vi "CSIRO XYZ Target Stage Control.vi"() -> ()   [LabVIEW 2018]
uses:
  PerformaxLV_v103.llb/commandsnew.ctl
  HYMOD MAIA/GLOBAL XYZ STAGE POSITION.vi
  Microdaq FPGA Development/USB XYZ Stage Reference.vi
panel:
  out "read_string 6":string
  out "read_string 5":string
  out "read_string 4":string
  out "DIVERGENCE 2":i32
  in  "Tab Control 3":T1(tab)=enum."CAL"
  in  "ENABLE MOTORS":bool
  in  "SPEED":i32(ring) items=["FAST", "NORMAL", "SLOW", "VERY SLOW", "ULTRASLOW"]
  in  "SET ZERO":bool
  out "Z":dbl[unit]=5.5500255e-05 caption="OY" format="%_6f"
  out "X":dbl[unit]=4.4501529999999996e-05 format="%_6f"
  out "Y":dbl[unit]=5.550153e-05 caption="OY" format="%_6f"
  in  "OY +":bool
  in  "OX -":bool
  in  "OX+":bool
  in  "OY-":bool
  in  "STOP":bool
  out "Y 2":bool
  out "X 2":bool
  out "Z":bool
  in  "DEFINED OBJECT":bool=TRUE
  in  "DEFINED LOCATIONS":i32(ring) items=["GLASS", "2000 CU GRID", "PHOSPHORUS", "5mm Aperture", "OPEN"]
  out "CURRENT LOCATION":string
  out "Z ENC":i32=1
  in  "Y B":dbl[unit] format="%_5f"
  in  "Y A":dbl[unit]=6.950000000000002e-08 format="%#_4f"
  in  "X B":dbl[unit] format="%_5f"
  in  "X A":dbl[unit]=6.950000000000001e-08 format="%#_4f"
  in  "MOVE OBJECT":T2 {"Z" format="%#_5f"; "Y" format="%#_5f"; "X" format="%#_5f"}
  in  "MOVE OBJECTS":bool
  out "X ENC":i32=6
  out "Y ENC":i32=6
  in  "Z A":dbl[unit]=2.5e-07 format="%#_4f"
  in  "Z B":dbl[unit] format="%_5f"
  in  "LOCATIONARRAY":T3(array[cluster])=[{"X"=0.063, "Y"=0.063, "DEFINITION"="0-1mm Object"}, {"X"=0.07602, "Y"=0.08773, "DEFINITION"="1mm Object"}, {"X"=0.08789, "Y"=0.07540000000000001, "DEFINITION"="2mm Object"}, {"X"=0.08789, "Y"=0.08773, "DEFINITION"="5mm Object"}, {"X"=0.12, "Y"=0.12, "DEFINITION"="10mm Object"}, {"X"=0.12, "Y"=0.10073, "DEFINITION"="OUT"}] {"Y" format="%#_4f"; "X" format="%#_4f"}
  in  "OHSPEED":i32=2000 min=1 max=400000 step=1
  in  "OLSPEED":i32=200 min=100 max=490550
  in  "OXACC":i32=300 min=1 max=5000
  in  "OYACC":i32=300 min=1 max=5000
  # "STOP"
  # "Calibration of Motor Positions"
  # "Aperture = A*enc step + B (mm)"
  # "NOTE: 1enc step = 2.5 * motor step"
  # "centre = red dot near 2nd thru hole\ngrid = +5mm (right), +15mm (up)\nsci = +8mm (right),  +13mm (up)\nglass =  +8mm (right), 0mm (up)"
  # "Speed Settings (pps)"
  # "Acceleration (ms)"
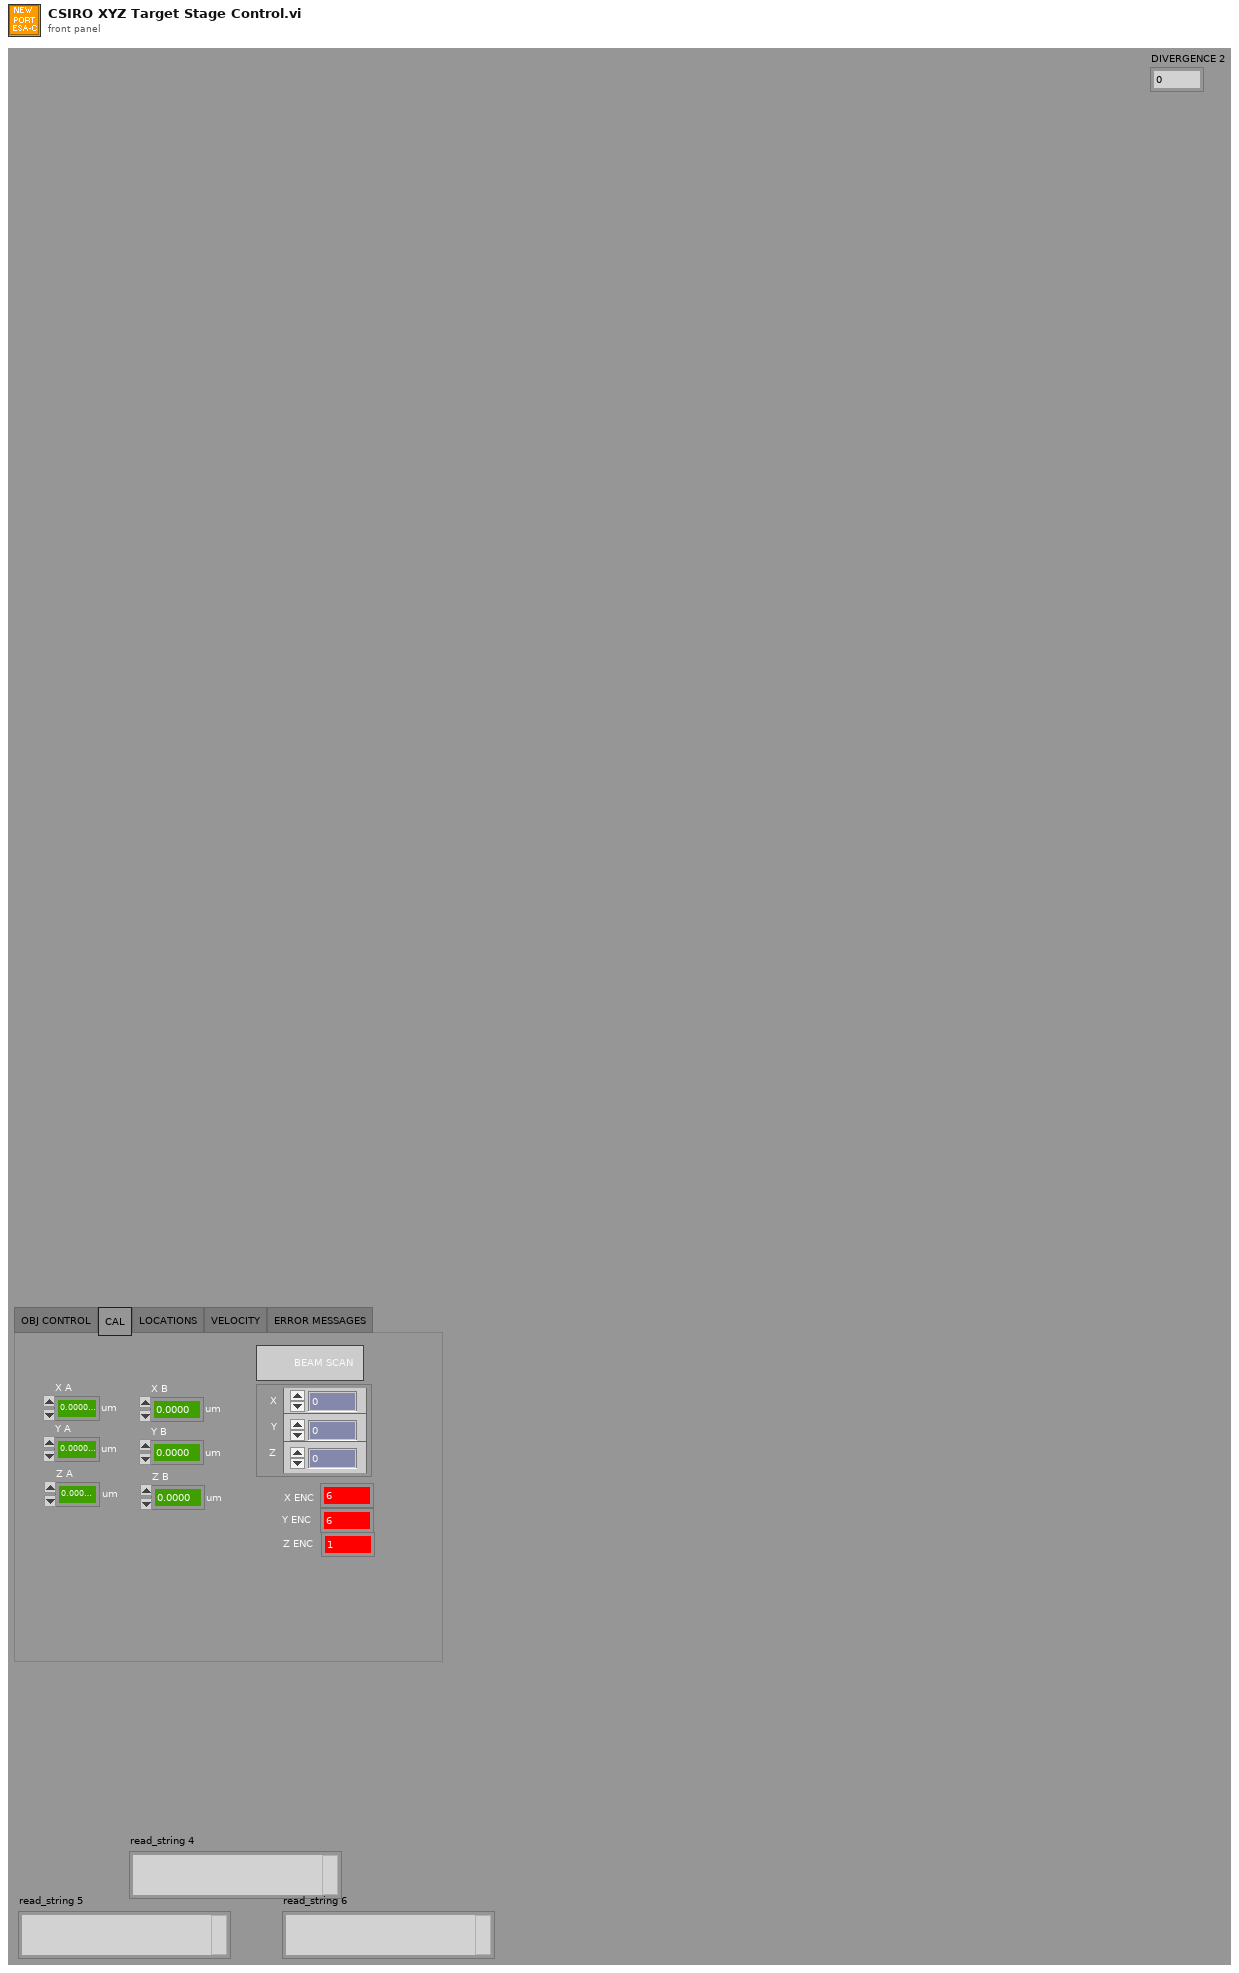
[diagram p1: front panel]
types:
  T1 = enum32{"OBJ CONTROL", "CAL", "LOCATIONS", "VELOCITY", "ERROR MESSAGES"}
  T2 = cluster{"X":dbl[unit], "Y":dbl[unit], "Z":dbl[unit]}
  T3 = cluster{"X":dbl[unit], "Y":dbl[unit], "DEFINITION":string}[]
  T4 = typedef "commandsnew.ctl" = enum16{"clearErr", "constJogNeg", "constJogPos", "getAccel", "getDeviceId", "getFirmwareVer", "getHighSpeed", "getIdleAmp", "getLowSpeed", "getMicroStep", "getMotorStatus", "getPolarity", "getPosition", "getProdId", "getPwrStatus", "getRunAmp", "getStatus", "getTemp", "homeNeg", "homePos", "moveToPosition", "powerDown", "powerUp", "setAccel", "setDeviceId", "setHighSpeed", "setIdleAmp", "setLowSpeed", "setMicroStep", "setPolarityLow", "setPolarityHigh", "setPosition", "setRunAmp", "stopFast", "stopSlow"}
  T5 = cluster{"X":dbl[unit], "Y":dbl[unit], "DEFINITION":string}
  T6 = cluster{"X":dbl[unit], "Y":dbl[unit], "CURRENT LOCATION":string}
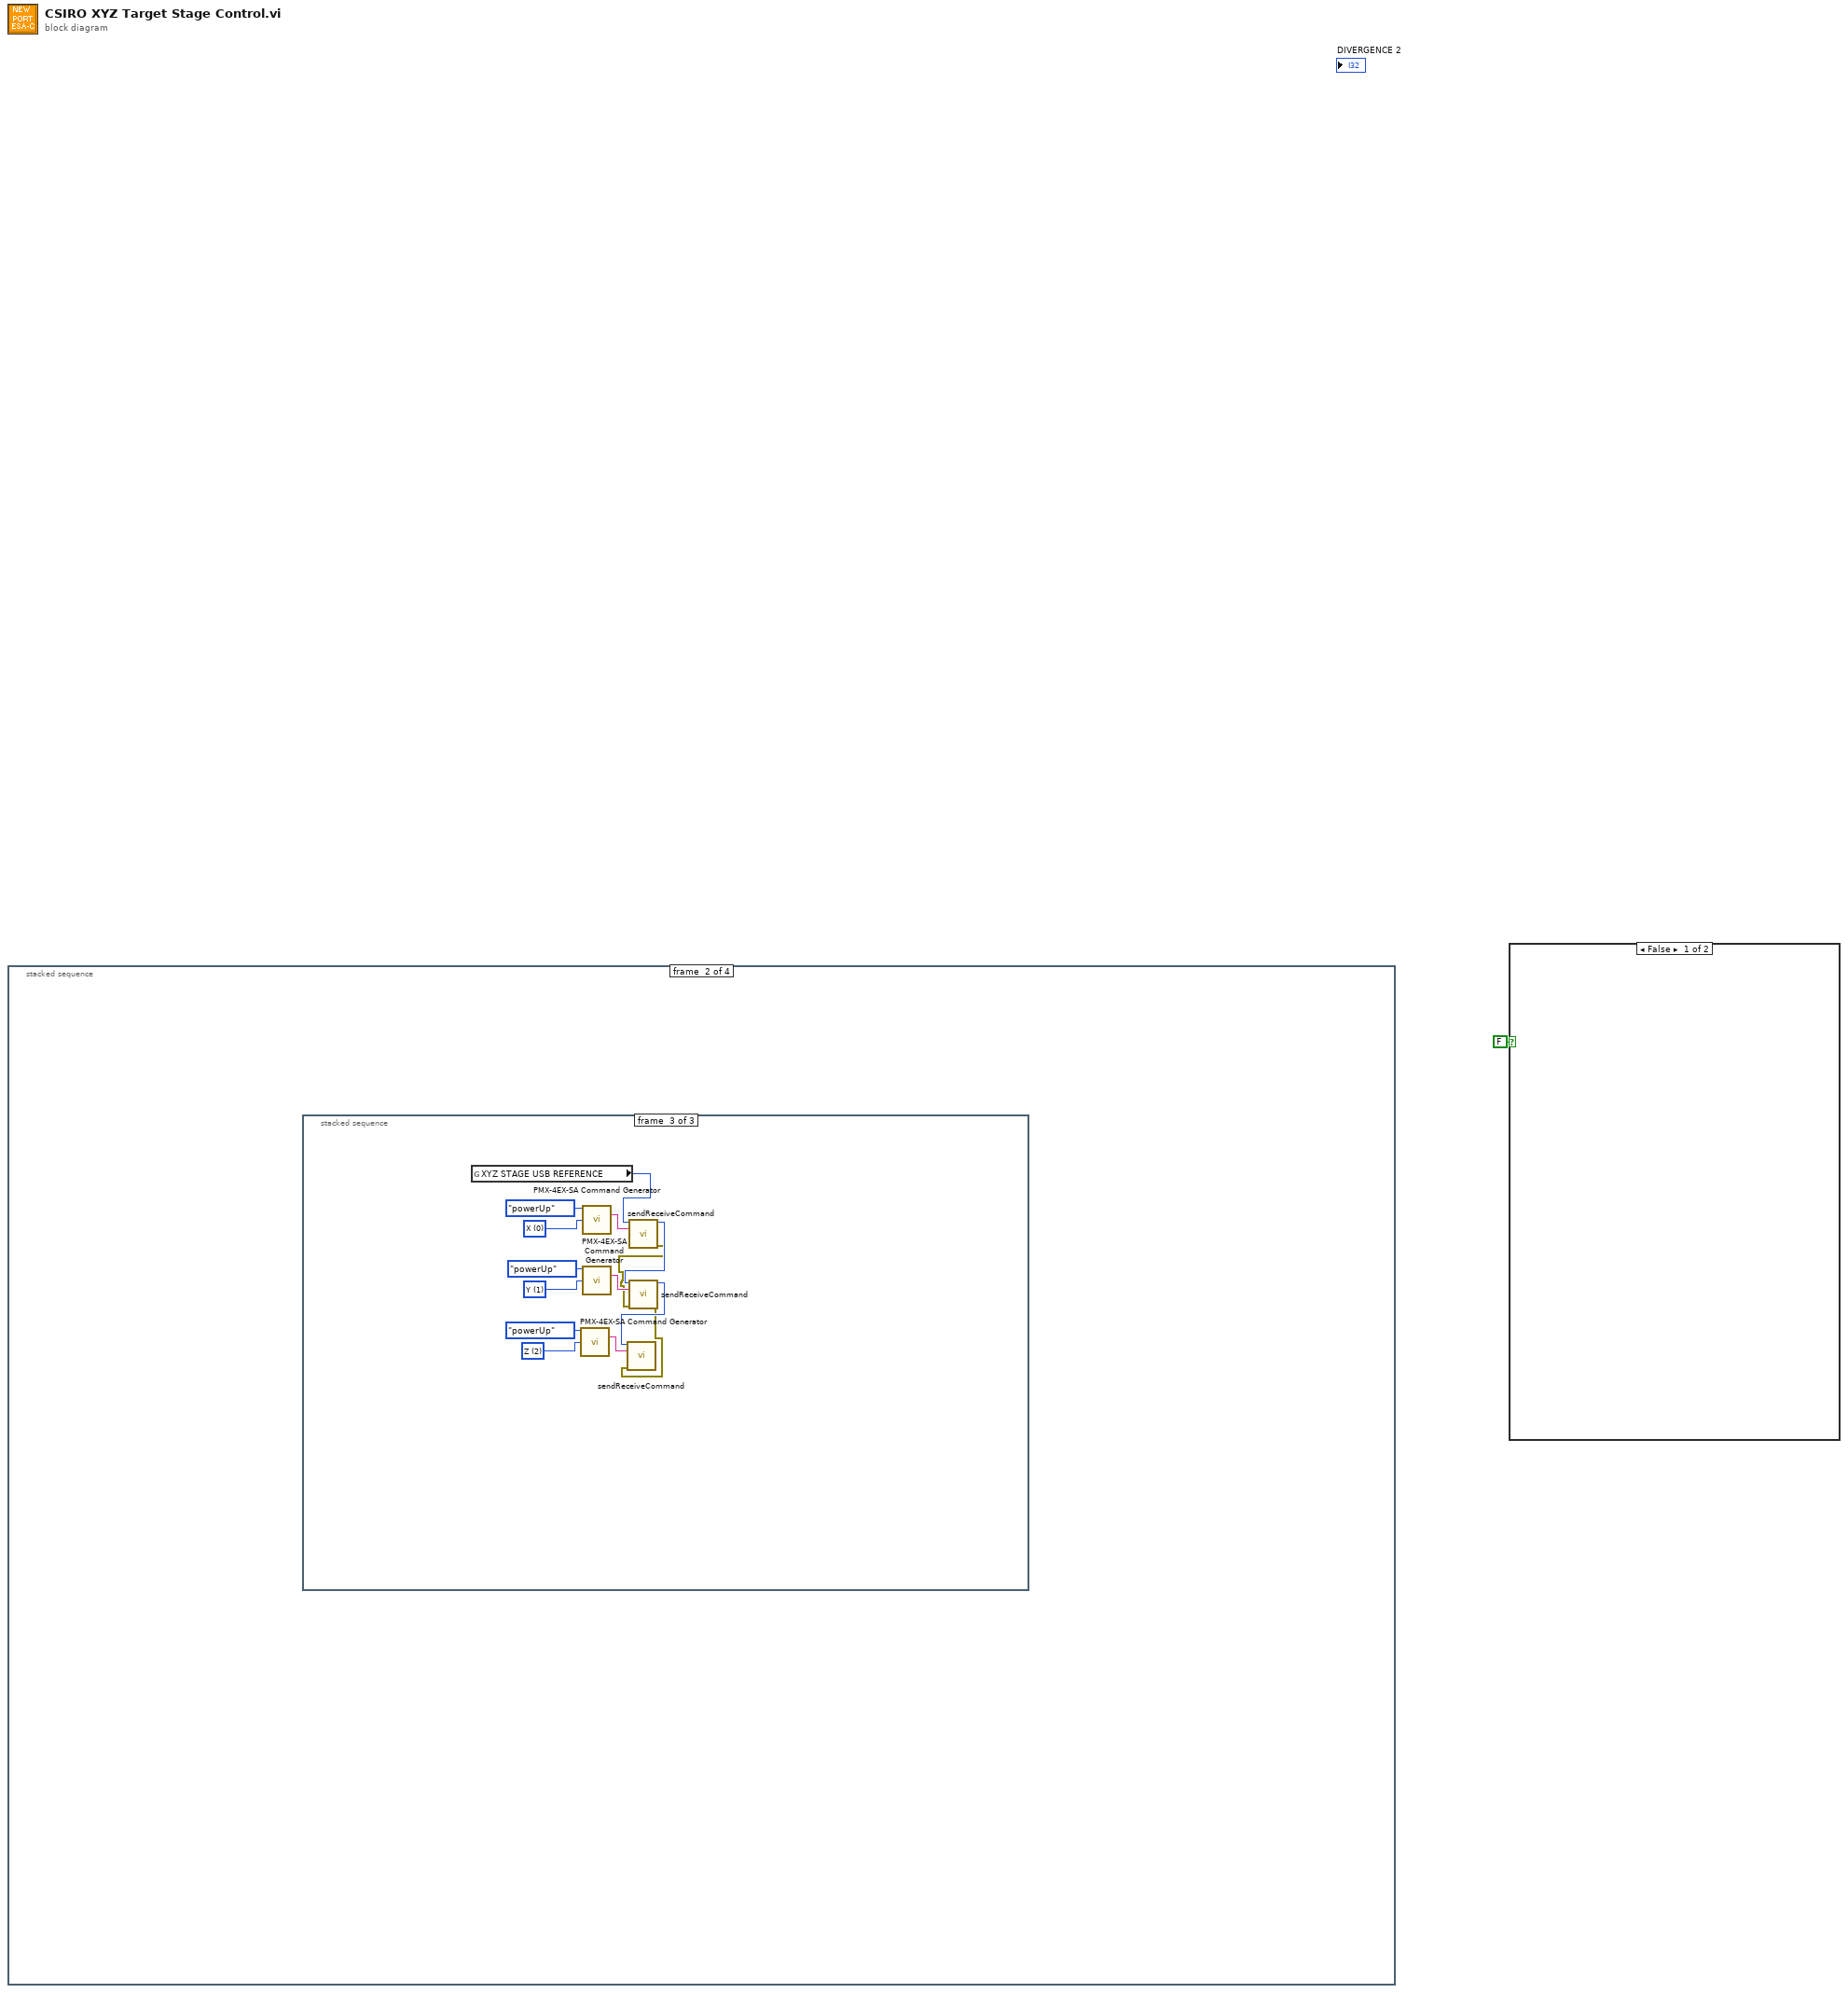
[diagram p0: block diagram]
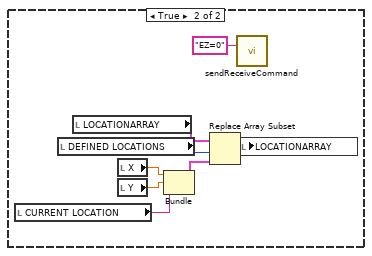
[diagram p2: hidden frame]
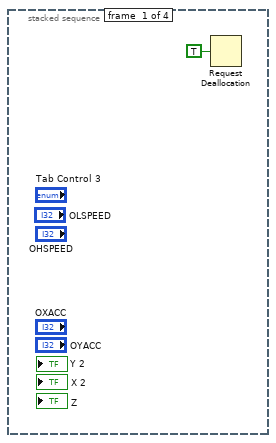
[diagram p3: hidden frame]
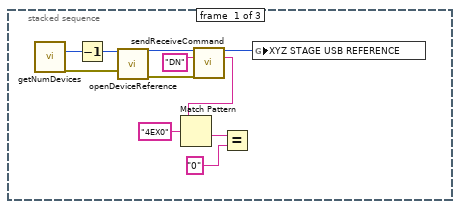
[diagram p4: hidden frame]
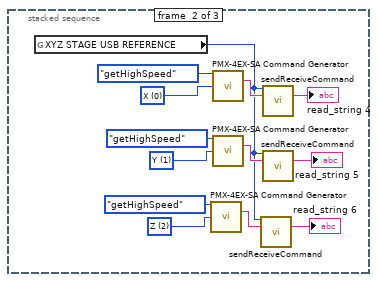
[diagram p5: hidden frame]
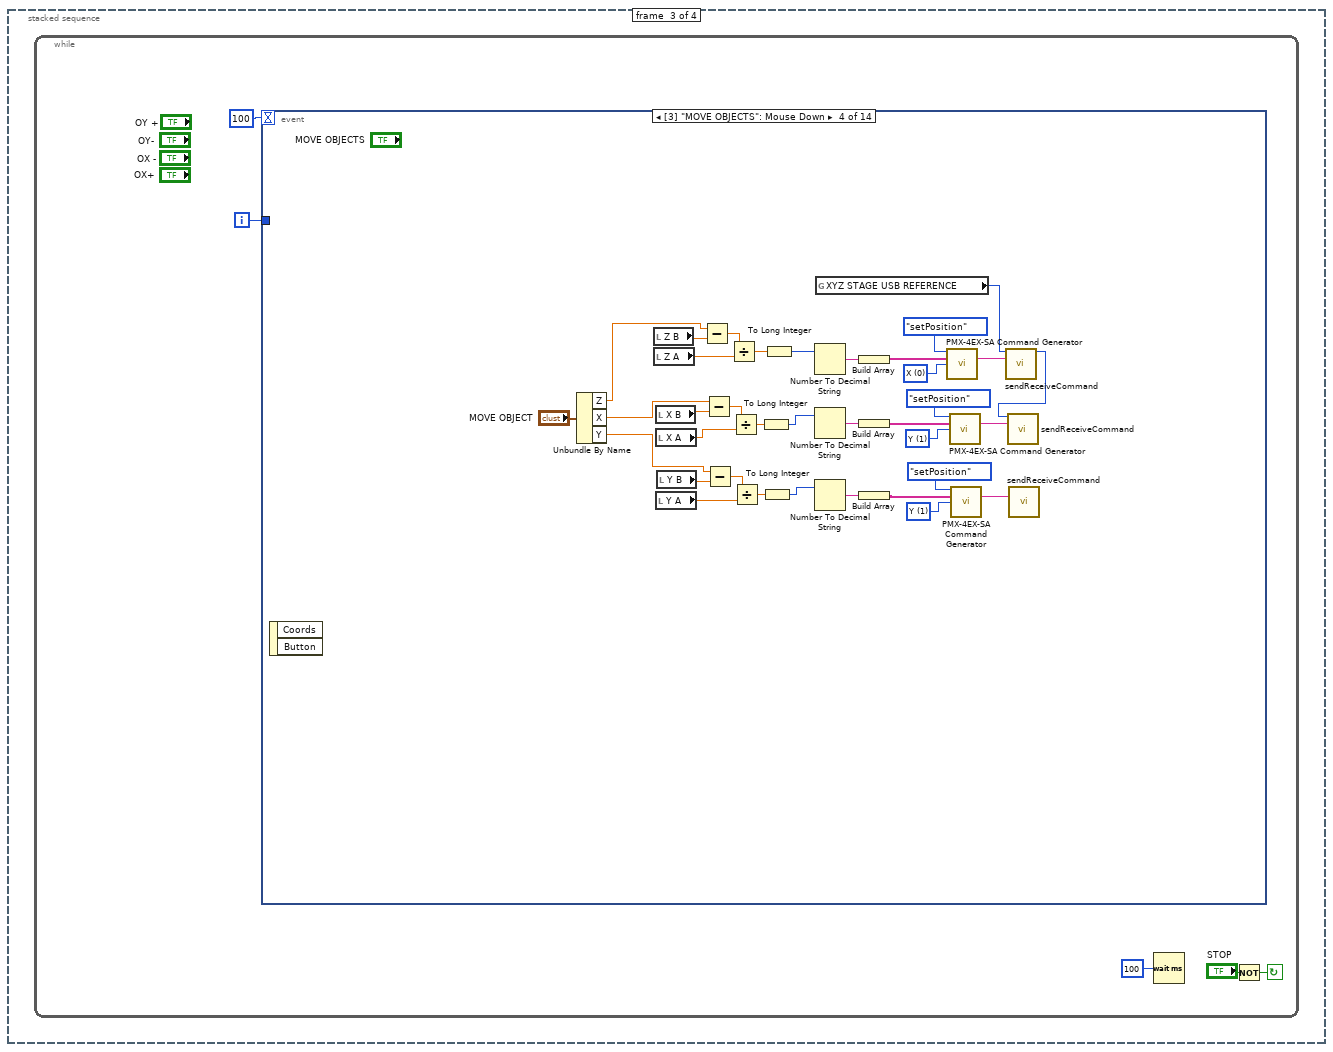
[diagram p6: hidden frame]
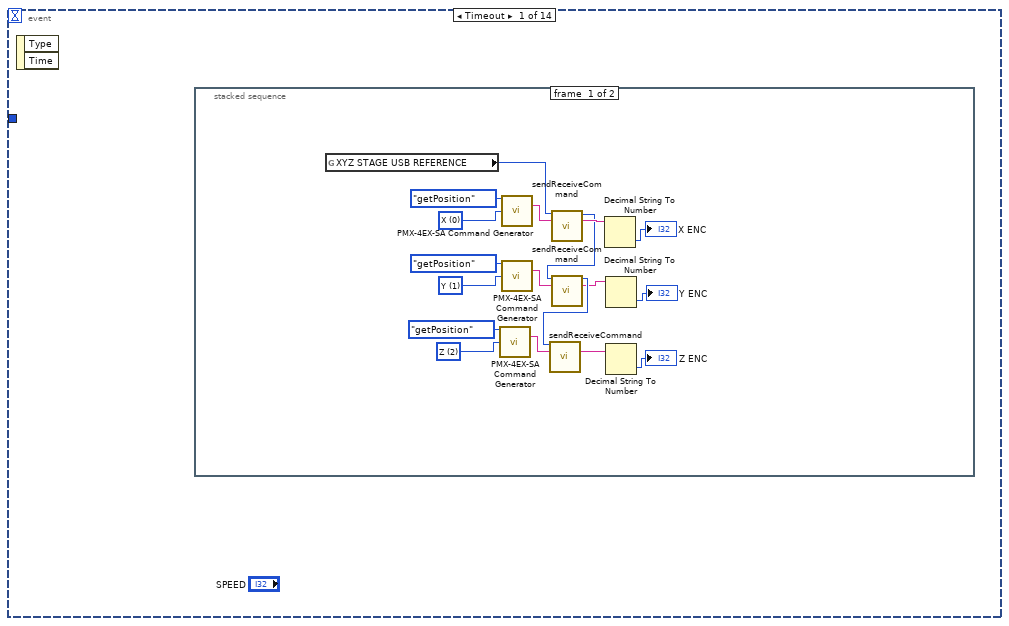
[diagram p7: hidden frame]
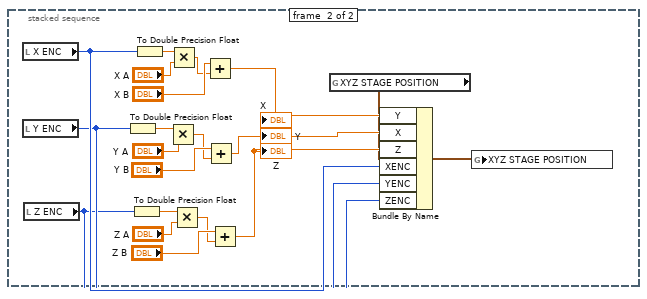
[diagram p8: hidden frame]
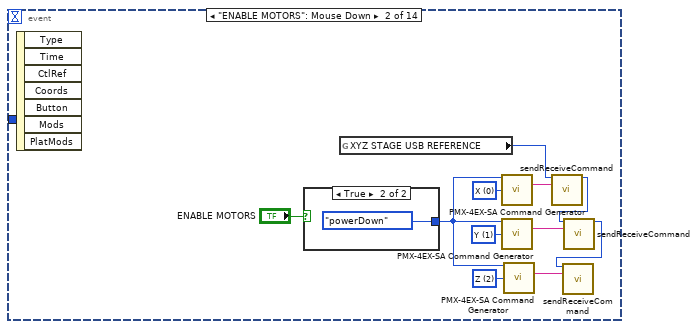
[diagram p9: hidden frame]
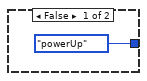
[diagram p10: hidden frame]
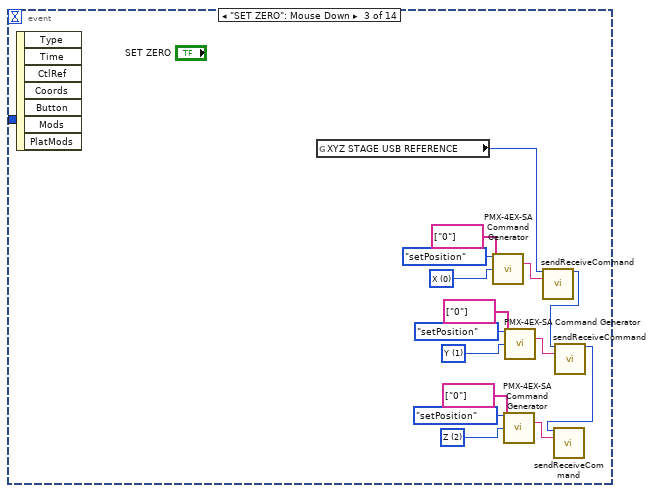
[diagram p11: hidden frame]
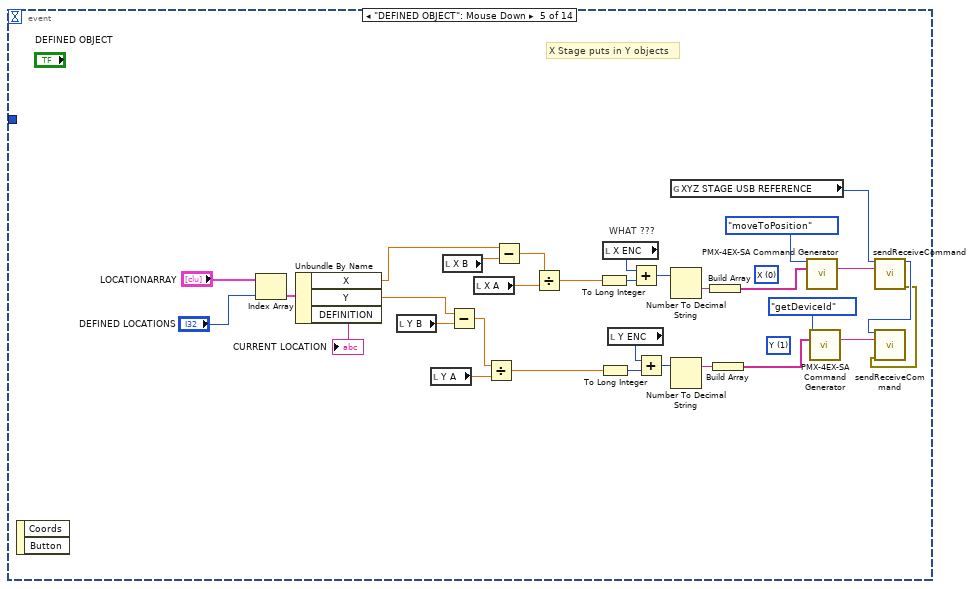
[diagram p12: hidden frame]
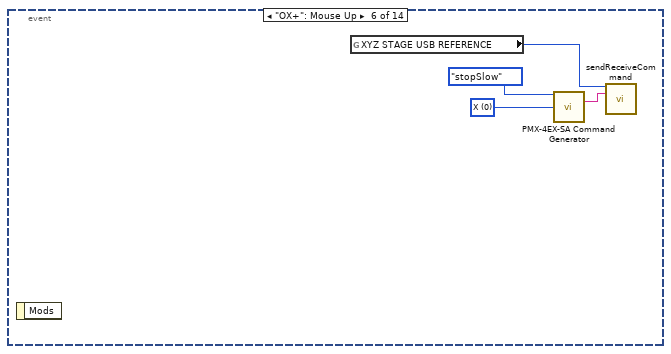
[diagram p13: hidden frame]
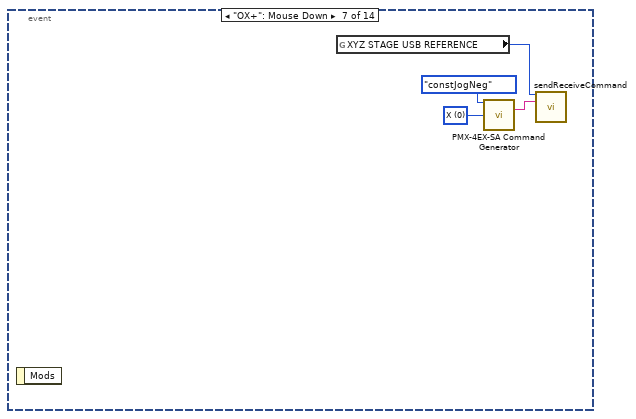
[diagram p14: hidden frame]
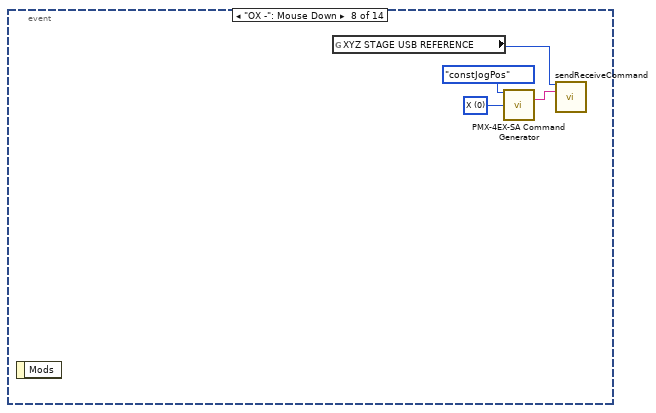
[diagram p15: hidden frame]
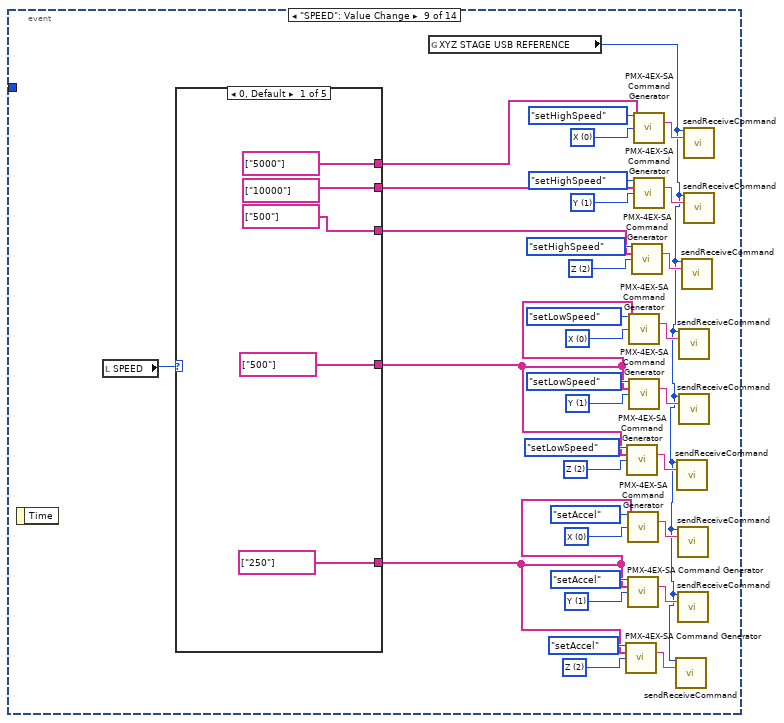
[diagram p16: hidden frame]
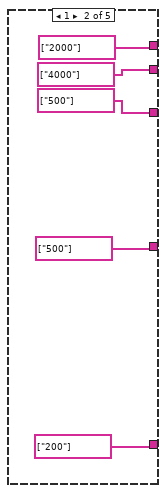
[diagram p17: hidden frame]
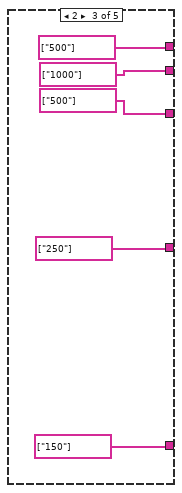
[diagram p18: hidden frame]
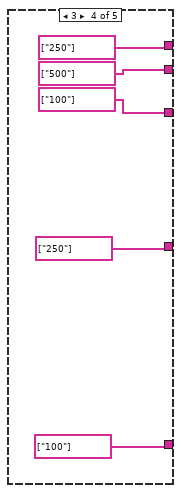
[diagram p19: hidden frame]
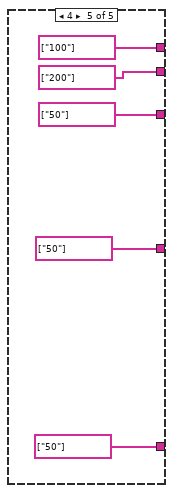
[diagram p20: hidden frame]
diagram:
  n1 = stacked-sequence {
    frame #0 {
      n2 = Request Deallocation(TRUE ("flag")) -> ()
    }
    frame #1 {
      n3 = stacked-sequence {
        frame #0 {
          n4 = call "getNumDevices.vi"() -> ("num_of_devices (out)"=w5:i32, "error out"=w13:errorcluster)  [unwired: 14 in]
          n5 = Decrement(x=w5) -> (x-1=w4:i32)
          n6 = call "openDeviceReference.vi"("deviceIndex"=w4, "error in (no error)"=w13) -> ("reference"=w12:i32, "error out"=w6:errorcluster)  [unwired: 12 in]
          n7 = call "sendReceiveCommand.vi"("reference (in)"=w12, "write_string"="DN", "error in (no error)"=w6) -> ("reference (out)"=w3:i32, "read_string"=w10:string)  [unwired: 10 in, 1 out]
          n8 = Match Pattern(string=w10, regular expression="4EX0") -> (after substring=w7:string)  [unwired: 1 in, 3 out]
          n9 = Equal?(x=w7, y="0") -> ()  [unwired: 1 out]
          n10 = global write "USB XYZ Stage Reference.vi" "XYZ STAGE USB REFERENCE"(w3) -> ()
        }
        frame #1 {
          w26 = u16 2 items=["X", "Y", "Z", "U"] ("AXIS")
          w23 = u16 1 items=["X", "Y", "Z", "U"] ("AXIS")
          w20 = u16 0 items=["X", "Y", "Z", "U"] ("AXIS")
          n11 = global read "USB XYZ Stage Reference.vi" "XYZ STAGE USB REFERENCE"() -> (w14:i32)
          n12 = call "PMX-4EX-SA Command Generator.vi"("COMMAND"=commandsnew."getHighSpeed", "AXIS"=w26) -> ("COMMAND"=w25:string)  [unwired: 13 in]
          n13 = call "PMX-4EX-SA Command Generator.vi"("COMMAND"=commandsnew."getHighSpeed", "AXIS"=w20) -> ("COMMAND"=w19:string)  [unwired: 13 in]
          n14 = call "PMX-4EX-SA Command Generator.vi"("COMMAND"=commandsnew."getHighSpeed", "AXIS"=w23) -> ("COMMAND"=w22:string)  [unwired: 13 in]
          n15 = call "sendReceiveCommand.vi"("reference (in)"=w14, "write_string"=w25) -> ("read_string"=→"read_string 6":string)  [unwired: 11 in, 2 out]
          n16 = call "sendReceiveCommand.vi"("reference (in)"=w14, "write_string"=w19) -> ("read_string"=→"read_string 4":string)  [unwired: 11 in, 2 out]
          n17 = call "sendReceiveCommand.vi"("reference (in)"=w14, "write_string"=w22) -> ("read_string"=→"read_string 5":string)  [unwired: 11 in, 2 out]
        }
        frame #2 {
          w32 = u16 2 items=["X", "Y", "Z", "U"] ("AXIS")
          w35 = u16 1 items=["X", "Y", "Z", "U"] ("AXIS")
          w38 = u16 0 items=["X", "Y", "Z", "U"] ("AXIS")
          n18 = global read "USB XYZ Stage Reference.vi" "XYZ STAGE USB REFERENCE"() -> (w27:i32)
          n19 = call "PMX-4EX-SA Command Generator.vi"("COMMAND"=commandsnew."powerUp", "AXIS"=w32) -> ("COMMAND"=w33:string)  [unwired: 13 in]
          n20 = call "PMX-4EX-SA Command Generator.vi"("COMMAND"=commandsnew."powerUp", "AXIS"=w38) -> ("COMMAND"=w39:string)  [unwired: 13 in]
          n21 = call "PMX-4EX-SA Command Generator.vi"("COMMAND"=commandsnew."powerUp", "AXIS"=w35) -> ("COMMAND"=w36:string)  [unwired: 13 in]
          n22 = call "sendReceiveCommand.vi"("reference (in)"=w27, "write_string"=w39) -> ("reference (out)"=w31:i32, "error out"=w29:errorcluster)  [unwired: 11 in, 1 out]
          n23 = call "sendReceiveCommand.vi"("reference (in)"=w31, "write_string"=w36, "error in (no error)"=w29) -> ("reference (out)"=w30:i32, "error out"=w28:errorcluster)  [unwired: 10 in, 1 out]
          n24 = call "sendReceiveCommand.vi"("reference (in)"=w30, "write_string"=w33, "error in (no error)"=w28) -> ()  [unwired: 10 in, 3 out]
        }
      }
    }
    frame #2 {
      n25 = while {
        i -> [w42]
        stop <- w44 continue-if-true
        n26 = event shown="[3] \"MOVE OBJECTS\": Mouse Down" {
          selector: _ -> [_ _ _ _ _ _ _ _ _ _ _ _ _ _]
          dyn-events: _ -> [_ _ _ _ _ _ _ _ _ _ _ _ _ _]
          timeout: 100 -> [_ _ _ _ _ _ _ _ _ _ _ _ _ _]
          tunnel: w42 -> [_ _ _ _ _ _ _ _ _ _ _ _ _ _]
          event Timeout {
            n27 = event-data() -> ()  [unwired: 3 out]
            n28 = stacked-sequence {
              frame #0 {
                w54 = u16 2 items=["X", "Y", "Z", "U"] ("AXIS")
                w57 = u16 1 items=["X", "Y", "Z", "U"] ("AXIS")
                w61 = u16 0 items=["X", "Y", "Z", "U"] ("AXIS")
                n29 = global read "USB XYZ Stage Reference.vi" "XYZ STAGE USB REFERENCE"() -> (w46:i32)
                n30 = call "PMX-4EX-SA Command Generator.vi"("COMMAND"=commandsnew."getPosition", "AXIS"=w54) -> ("COMMAND"=w55:string)  [unwired: 13 in]
                n31 = call "PMX-4EX-SA Command Generator.vi"("COMMAND"=commandsnew."getPosition", "AXIS"=w61) -> ("COMMAND"=w62:string)  [unwired: 13 in]
                n32 = call "PMX-4EX-SA Command Generator.vi"("COMMAND"=commandsnew."getPosition", "AXIS"=w57) -> ("COMMAND"=w58:string)  [unwired: 13 in]
                n33 = call "sendReceiveCommand.vi"("reference (in)"=w46, "write_string"=w62) -> ("reference (out)"=w53:i32, "read_string"=w60:string)  [unwired: 11 in, 1 out]
                n34 = call "sendReceiveCommand.vi"("reference (in)"=w53, "write_string"=w58) -> ("reference (out)"=w52:i32, "read_string"=w51:string)  [unwired: 11 in, 1 out]
                n35 = call "sendReceiveCommand.vi"("reference (in)"=w52, "write_string"=w55) -> ("read_string"=w50:string)  [unwired: 11 in, 2 out]
                n36 = Decimal String To Number(string=w60) -> (number=→"X ENC":i32)  [unwired: 2 in, 1 out]
                n37 = Decimal String To Number(string=w51) -> (number=→"Y ENC":i32)  [unwired: 2 in, 1 out]
                n38 = Decimal String To Number(string=w50) -> (number=→"Z ENC":i32)  [unwired: 2 in, 1 out]
              }
              frame #1 {
                n39 = local read "X ENC"() -> (w66:i32)
                n40 = local read "Y ENC"() -> (w65:i32)
                n41 = local read "Z ENC"() -> (w64:i32)
                n42 = To Double Precision Float(number=w65) -> (double precision float=w76:dbl)
                n43 = To Double Precision Float(number=w64) -> (double precision float=w72:dbl)
                n44 = To Double Precision Float(number=w66) -> (double precision float=w81:dbl)
                n45 = Multiply(x=w76, y="Y A") -> (x*y=w78:dbl[unit])
                n46 = Multiply(x=w81, y="X A") -> (x*y=w82:dbl[unit])
                n47 = Multiply(x=w72, y="Z A") -> (x*y=w74:dbl[unit])
                n48 = Add(x="X B", y=w82) -> (x+y=w71:dbl[unit])
                "X" <- w71
                n49 = Add(x="Y B", y=w78) -> (x+y=w70:dbl[unit])
                "Y" <- w70
                n50 = Add(x="Z B", y=w74) -> (x+y=w69:dbl[unit])
                "Z" <- w69
                n51 = global read "GLOBAL XYZ STAGE POSITION.vi" "XYZ STAGE POSITION"() -> (w68:T2)
                n52 = Bundle By Name(cluster=w68, "Y"=w71, "X"=w70, "Z"=w69, "XENC"=w66, "YENC"=w65, "ZENC"=w64) -> (w67:T2)
                n53 = global write "GLOBAL XYZ STAGE POSITION.vi" "XYZ STAGE POSITION"(w67) -> ()
              }
            }
          }
          event "ENABLE MOTORS": Mouse Down {
            w90 = u16 2 items=["X", "Y", "Z", "U"] ("AXIS")
            w92 = u16 1 items=["X", "Y", "Z", "U"] ("AXIS")
            w94 = u16 0 items=["X", "Y", "Z", "U"] ("AXIS")
            n54 = event-data() -> ()  [unwired: 8 out]
            n55 = case shown="True" "ENABLE MOTORS" {
              tunnel: [commandsnew."powerUp" ("COMMAND") commandsnew."powerDown" ("COMMAND")] -> w86
              frame False {
              }
              frame True {
              }
            }
            n56 = global read "USB XYZ Stage Reference.vi" "XYZ STAGE USB REFERENCE"() -> (w84:i32)
            n57 = call "PMX-4EX-SA Command Generator.vi"("COMMAND"=w86, "AXIS"=w94) -> ("COMMAND"=w93:string)  [unwired: 13 in]
            n58 = call "PMX-4EX-SA Command Generator.vi"("COMMAND"=w86, "AXIS"=w92) -> ("COMMAND"=w91:string)  [unwired: 13 in]
            n59 = call "PMX-4EX-SA Command Generator.vi"("COMMAND"=w86, "AXIS"=w90) -> ("COMMAND"=w89:string)  [unwired: 13 in]
            n60 = call "sendReceiveCommand.vi"("reference (in)"=w84, "write_string"=w93) -> ("reference (out)"=w88:i32)  [unwired: 11 in, 2 out]
            n61 = call "sendReceiveCommand.vi"("reference (in)"=w88, "write_string"=w91) -> ("reference (out)"=w87:i32)  [unwired: 11 in, 2 out]
            n62 = call "sendReceiveCommand.vi"("reference (in)"=w87, "write_string"=w89) -> ()  [unwired: 11 in, 3 out]
          }
          event "SET ZERO": Mouse Down {
            w102 = u16 2 items=["X", "Y", "Z", "U"] ("AXIS")
            w106 = u16 1 items=["X", "Y", "Z", "U"] ("AXIS")
            w110 = u16 0 items=["X", "Y", "Z", "U"] ("AXIS")
            n63 = event-data() -> ()  [unwired: 8 out]
            n64 = global read "USB XYZ Stage Reference.vi" "XYZ STAGE USB REFERENCE"() -> (w97:i32)
            n65 = call "PMX-4EX-SA Command Generator.vi"("COMMAND"=commandsnew."setPosition", "args"=string[] ["0"], "AXIS"=w110) -> ("COMMAND"=w109:string)  [unwired: 12 in]
            n66 = call "PMX-4EX-SA Command Generator.vi"("COMMAND"=commandsnew."setPosition", "args"=string[] ["0"], "AXIS"=w102) -> ("COMMAND"=w101:string)  [unwired: 12 in]
            n67 = call "PMX-4EX-SA Command Generator.vi"("COMMAND"=commandsnew."setPosition", "args"=string[] ["0"], "AXIS"=w106) -> ("COMMAND"=w105:string)  [unwired: 12 in]
            n68 = call "sendReceiveCommand.vi"("reference (in)"=w97, "write_string"=w109) -> ("reference (out)"=w99:i32)  [unwired: 11 in, 2 out]
            n69 = call "sendReceiveCommand.vi"("reference (in)"=w99, "write_string"=w105) -> ("reference (out)"=w98:i32)  [unwired: 11 in, 2 out]
            n70 = call "sendReceiveCommand.vi"("reference (in)"=w98, "write_string"=w101) -> ()  [unwired: 11 in, 3 out]
          }
          event "MOVE OBJECTS": Mouse Down {
            w116 = u16 1 items=["X", "Y", "Z", "U"] ("AXIS")
            w136 = u16 1 items=["X", "Y", "Z", "U"] ("AXIS")
            w137 = u16 0 items=["X", "Y", "Z", "U"] ("AXIS")
            n71 = event-data() -> ()  [unwired: 3 out]
            n72 = Unbundle By Name("MOVE OBJECT") -> ("Z"=w127:dbl[unit], "X"=w126:dbl[unit], "Y"=w125:dbl[unit])
            n73 = local read "Z B"() -> (w124:dbl[unit])
            n74 = local read "Z A"() -> (w135:dbl[unit])
            n75 = local read "X B"() -> (w122:dbl[unit])
            n76 = local read "X A"() -> (w131:dbl[unit])
            n77 = local read "Y A"() -> (w133:dbl[unit])
            n78 = local read "Y B"() -> (w123:dbl[unit])
            n79 = Subtract(x=w127, y=w124) -> (x-y=w134:dbl[unit])
            n80 = Subtract(x=w126, y=w122) -> (x-y=w130:dbl[unit])
            n81 = Subtract(x=w125, y=w123) -> (x-y=w132:dbl[unit])
            n82 = Divide(x=w134, y=w135) -> (x/y=w119:dbl)
            n83 = Divide(x=w130, y=w131) -> (x/y=w120:dbl)
            n84 = Divide(x=w132, y=w133) -> (x/y=w121:dbl)
            n85 = To Long Integer(number=w120) -> (32bit integer=w128:i32)
            n86 = To Long Integer(number=w121) -> (32bit integer=w115:i32)
            n87 = To Long Integer(number=w119) -> (32bit integer=w129:i32)
            n88 = Number To Decimal String(number=w129) -> (decimal integer string=w146:string)  [unwired: 1 out]
            n89 = Number To Decimal String(number=w128) -> (decimal integer string=w147:string)  [unwired: 1 out]
            n90 = Number To Decimal String(number=w115) -> (decimal integer string=w114:string)  [unwired: 1 out]
            n91 = global read "USB XYZ Stage Reference.vi" "XYZ STAGE USB REFERENCE"() -> (w112:i32)
            n92 = Build Array(w146) -> (w144:string[])
            n93 = Build Array(w147) -> (w143:string[])
            n94 = Build Array(w114) -> (w113:string[])
            n95 = call "PMX-4EX-SA Command Generator.vi"("COMMAND"=commandsnew."setPosition" ("commands"), "args"=w144, "AXIS"=w137) -> ("COMMAND"=w142:string)  [unwired: 12 in]
            n96 = call "PMX-4EX-SA Command Generator.vi"("COMMAND"=commandsnew."setPosition" ("commands"), "args"=w143, "AXIS"=w136) -> ("COMMAND"=w140:string)  [unwired: 12 in]
            n97 = call "PMX-4EX-SA Command Generator.vi"("COMMAND"=commandsnew."setPosition" ("commands"), "args"=w113, "AXIS"=w116) -> ("COMMAND"=w118:string)  [unwired: 12 in]
            n98 = call "sendReceiveCommand.vi"("reference (in)"=w112, "write_string"=w142) -> ("reference (out)"=w138:i32)  [unwired: 11 in, 2 out]
            n99 = call "sendReceiveCommand.vi"("reference (in)"=w138, "write_string"=w140) -> ()  [unwired: 11 in, 3 out]
            n100 = call "sendReceiveCommand.vi"("write_string"=w118) -> ()  [unwired: 12 in, 3 out]
          }
          event "DEFINED OBJECT": Mouse Down {
            (unwired) u16 1 items=["X", "Y", "Z", "U"] ("AXIS")
            (unwired) u16 0 items=["X", "Y", "Z", "U"] ("AXIS")
            # "WHAT ???"
            # "X Stage puts in Y objects"
            n101 = event-data() -> ()  [unwired: 3 out]
            n102 = Index Array(array="LOCATIONARRAY", index="DEFINED LOCATIONS") -> (element=w166:T5)
            n103 = Unbundle By Name(w166) -> ("X"=w158:dbl[unit], "Y"=w157:dbl[unit], "DEFINITION"=→"CURRENT LOCATION":string)
            n104 = local read "Y B"() -> (w163:dbl[unit])
            n105 = local read "Y A"() -> (w164:dbl[unit])
            n106 = local read "X B"() -> (w160:dbl[unit])
            n107 = Subtract(x=w157, y=w163) -> (x-y=w162:dbl[unit])
            n108 = local read "X A"() -> (w159:dbl[unit])
            n109 = Divide(x=w162, y=w164) -> (x/y=w149:dbl)
            n110 = Subtract(x=w158, y=w160) -> (x-y=w161:dbl[unit])
            n111 = Divide(x=w161, y=w159) -> (x/y=w150:dbl)
            n112 = To Long Integer(number=w150) -> (32bit integer=w155:i32)
            n113 = To Long Integer(number=w149) -> (32bit integer=w152:i32)
            n114 = local read "X ENC"() -> (w156:i32)
            n115 = local read "Y ENC"() -> (w153:i32)
            n116 = Add(x=w156, y=w155) -> (x+y=w154:i32)
            n117 = Add(x=w153, y=w152) -> (x+y=w151:i32)
            n118 = global read "USB XYZ Stage Reference.vi" "XYZ STAGE USB REFERENCE"() -> (w148:i32)
            n119 = Number To Decimal String(number=w154) -> (decimal integer string=w173:string)  [unwired: 1 in]
            n120 = Number To Decimal String(number=w151) -> (decimal integer string=w171:string)  [unwired: 1 in]
            n121 = Build Array(w173) -> (w172:string[])
            n122 = Build Array(w171) -> (w170:string[])
            n123 = call "PMX-4EX-SA Command Generator.vi"("COMMAND"=commandsnew."moveToPosition" ("commands"), "args"=w172) -> ("COMMAND"=w178:string)  [unwired: 13 in]
            n124 = call "PMX-4EX-SA Command Generator.vi"("COMMAND"=commandsnew."getDeviceId" ("commands"), "args"=w170) -> ("COMMAND"=w176:string)  [unwired: 13 in]
            n125 = call "sendReceiveCommand.vi"("reference (in)"=w148, "write_string"=w178) -> ("reference (out)"=w174:i32, "error out"=w169:errorcluster)  [unwired: 11 in, 1 out]
            n126 = call "sendReceiveCommand.vi"("reference (in)"=w174, "write_string"=w176, "error in (no error)"=w169) -> ()  [unwired: 10 in, 3 out]
          }
          event "OX+": Mouse Up {
            w180 = u16 0 items=["X", "Y", "Z", "U"] ("AXIS")
            n127 = event-data() -> ()  [unwired: 2 out]
            n128 = global read "USB XYZ Stage Reference.vi" "XYZ STAGE USB REFERENCE"() -> (w179:i32)
            n129 = call "PMX-4EX-SA Command Generator.vi"("COMMAND"=commandsnew."stopSlow" ("commands"), "AXIS"=w180) -> ("COMMAND"=w182:string)  [unwired: 13 in]
            n130 = call "sendReceiveCommand.vi"("reference (in)"=w179, "write_string"=w182) -> ()  [unwired: 11 in, 3 out]
          }
          event "OX+": Mouse Down {
            w184 = u16 0 items=["X", "Y", "Z", "U"] ("AXIS")
            n131 = event-data() -> ()  [unwired: 2 out]
            n132 = global read "USB XYZ Stage Reference.vi" "XYZ STAGE USB REFERENCE"() -> (w183:i32)
            n133 = call "PMX-4EX-SA Command Generator.vi"("COMMAND"=commandsnew."constJogNeg" ("commands"), "AXIS"=w184) -> ("COMMAND"=w185:string)  [unwired: 13 in]
            n134 = call "sendReceiveCommand.vi"("reference (in)"=w183, "write_string"=w185) -> ()  [unwired: 11 in, 3 out]
          }
          event "OX -": Mouse Down {
            w188 = u16 0 items=["X", "Y", "Z", "U"] ("AXIS")
            n135 = event-data() -> ()  [unwired: 2 out]
            n136 = global read "USB XYZ Stage Reference.vi" "XYZ STAGE USB REFERENCE"() -> (w187:i32)
            n137 = call "PMX-4EX-SA Command Generator.vi"("COMMAND"=commandsnew."constJogPos" ("commands"), "AXIS"=w188) -> ("COMMAND"=w189:string)  [unwired: 13 in]
            n138 = call "sendReceiveCommand.vi"("reference (in)"=w187, "write_string"=w189) -> ()  [unwired: 11 in, 3 out]
          }
          event "SPEED": Value Change {
            w205 = u16 2 items=["X", "Y", "Z", "U"] ("AXIS")
            w202 = u16 1 items=["X", "Y", "Z", "U"] ("AXIS")
            w199 = u16 0 items=["X", "Y", "Z", "U"] ("AXIS")
            w214 = u16 2 items=["X", "Y", "Z", "U"] ("AXIS")
            w211 = u16 1 items=["X", "Y", "Z", "U"] ("AXIS")
            w208 = u16 0 items=["X", "Y", "Z", "U"] ("AXIS")
            w223 = u16 2 items=["X", "Y", "Z", "U"] ("AXIS")
            w220 = u16 1 items=["X", "Y", "Z", "U"] ("AXIS")
            w217 = u16 0 items=["X", "Y", "Z", "U"] ("AXIS")
            n139 = event-data() -> ()  [unwired: 2 out]
            n140 = local read "SPEED"() -> (w224:i32)
            n141 = case shown="0, Default" w224 {
              tunnel: [string[] ["5000"] ("args") string[] ["2000"] ("args") string[] ["500"] ("args") string[] ["250"] ("args") string[] ["100"] ("args")] -> w196
              tunnel: [string[] ["500"] ("args") string[] ["500"] ("args") string[] ["250"] ("args") string[] ["250"] ("args") string[] ["50"] ("args")] -> w195
              tunnel: [string[] ["250"] ("args") string[] ["200"] ("args") string[] ["150"] ("args") string[] ["100"] ("args") string[] ["50"] ("args")] -> w194
              tunnel: [string[] ["10000"] ("args") string[] ["4000"] ("args") string[] ["1000"] ("args") string[] ["500"] ("args") string[] ["200"] ("args")] -> w193
              tunnel: [string[] ["500"] ("args") string[] ["500"] ("args") string[] ["500"] ("args") string[] ["100"] ("args") string[] ["50"] ("args")] -> w192
              frame 0, Default {
              }
              frame 1 {
              }
              frame 2 {
              }
              frame 3 {
              }
              frame 4 {
              }
            }
            n142 = global read "USB XYZ Stage Reference.vi" "XYZ STAGE USB REFERENCE"() -> (w191:i32)
            n143 = call "PMX-4EX-SA Command Generator.vi"("COMMAND"=commandsnew."setAccel", "args"=w194, "AXIS"=w205) -> ("COMMAND"=w204:string)  [unwired: 12 in]
            n144 = call "PMX-4EX-SA Command Generator.vi"("COMMAND"=commandsnew."setLowSpeed", "args"=w195, "AXIS"=w214) -> ("COMMAND"=w213:string)  [unwired: 12 in]
            n145 = call "PMX-4EX-SA Command Generator.vi"("COMMAND"=commandsnew."setAccel", "args"=w194, "AXIS"=w199) -> ("COMMAND"=w198:string)  [unwired: 12 in]
            n146 = call "PMX-4EX-SA Command Generator.vi"("COMMAND"=commandsnew."setAccel", "args"=w194, "AXIS"=w202) -> ("COMMAND"=w201:string)  [unwired: 12 in]
            n147 = call "PMX-4EX-SA Command Generator.vi"("COMMAND"=commandsnew."setLowSpeed", "args"=w195, "AXIS"=w208) -> ("COMMAND"=w207:string)  [unwired: 12 in]
            n148 = call "PMX-4EX-SA Command Generator.vi"("COMMAND"=commandsnew."setLowSpeed", "args"=w195, "AXIS"=w211) -> ("COMMAND"=w210:string)  [unwired: 12 in]
            n149 = call "PMX-4EX-SA Command Generator.vi"("COMMAND"=commandsnew."setHighSpeed", "args"=w192, "AXIS"=w223) -> ("COMMAND"=w222:string)  [unwired: 12 in]
            n150 = call "PMX-4EX-SA Command Generator.vi"("COMMAND"=commandsnew."setHighSpeed", "args"=w196, "AXIS"=w217) -> ("COMMAND"=w216:string)  [unwired: 12 in]
            n151 = call "PMX-4EX-SA Command Generator.vi"("COMMAND"=commandsnew."setHighSpeed", "args"=w193, "AXIS"=w220) -> ("COMMAND"=w219:string)  [unwired: 12 in]
            n152 = call "sendReceiveCommand.vi"("reference (in)"=w191, "write_string"=w204) -> ()  [unwired: 11 in, 3 out]
            n153 = call "sendReceiveCommand.vi"("reference (in)"=w191, "write_string"=w213) -> ()  [unwired: 11 in, 3 out]
            n154 = call "sendReceiveCommand.vi"("reference (in)"=w191, "write_string"=w198) -> ()  [unwired: 11 in, 3 out]
            n155 = call "sendReceiveCommand.vi"("reference (in)"=w191, "write_string"=w201) -> ()  [unwired: 11 in, 3 out]
            n156 = call "sendReceiveCommand.vi"("reference (in)"=w191, "write_string"=w207) -> ()  [unwired: 11 in, 3 out]
            n157 = call "sendReceiveCommand.vi"("reference (in)"=w191, "write_string"=w210) -> ()  [unwired: 11 in, 3 out]
            n158 = call "sendReceiveCommand.vi"("reference (in)"=w191, "write_string"=w222) -> ()  [unwired: 11 in, 3 out]
            n159 = call "sendReceiveCommand.vi"("reference (in)"=w191, "write_string"=w216) -> ()  [unwired: 11 in, 3 out]
            n160 = call "sendReceiveCommand.vi"("reference (in)"=w191, "write_string"=w219) -> ()  [unwired: 11 in, 3 out]
          }
          event "OX -": Mouse Up {
            w252 = u16 0 items=["X", "Y", "Z", "U"] ("AXIS")
            n161 = event-data() -> ()  [unwired: 2 out]
            n162 = global read "USB XYZ Stage Reference.vi" "XYZ STAGE USB REFERENCE"() -> (w250:i32)
            n163 = call "PMX-4EX-SA Command Generator.vi"("COMMAND"=commandsnew."stopSlow" ("commands"), "AXIS"=w252) -> ("COMMAND"=w253:string)  [unwired: 13 in]
            n164 = call "sendReceiveCommand.vi"("reference (in)"=w250, "write_string"=w253) -> ()  [unwired: 11 in, 3 out]
          }
          event "OY +": Mouse Down {
            w255 = u16 1 items=["X", "Y", "Z", "U"] ("AXIS")
            n165 = event-data() -> ()  [unwired: 2 out]
            n166 = global read "USB XYZ Stage Reference.vi" "XYZ STAGE USB REFERENCE"() -> (w254:i32)
            n167 = call "PMX-4EX-SA Command Generator.vi"("COMMAND"=commandsnew."constJogNeg" ("commands"), "AXIS"=w255) -> ("COMMAND"=w256:string)  [unwired: 13 in]
            n168 = call "sendReceiveCommand.vi"("reference (in)"=w254, "write_string"=w256) -> ()  [unwired: 11 in, 3 out]
          }
          event "OY +": Mouse Up {
            w259 = u16 1 items=["X", "Y", "Z", "U"] ("AXIS")
            n169 = event-data() -> ()  [unwired: 2 out]
            n170 = global read "USB XYZ Stage Reference.vi" "XYZ STAGE USB REFERENCE"() -> (w258:i32)
            n171 = call "PMX-4EX-SA Command Generator.vi"("COMMAND"=commandsnew."stopSlow" ("commands"), "AXIS"=w259) -> ("COMMAND"=w261:string)  [unwired: 13 in]
            n172 = call "sendReceiveCommand.vi"("reference (in)"=w258, "write_string"=w261) -> ()  [unwired: 11 in, 3 out]
          }
          event "OY-": Mouse Down {
            w263 = u16 1 items=["X", "Y", "Z", "U"] ("AXIS")
            n173 = event-data() -> ()  [unwired: 2 out]
            n174 = global read "USB XYZ Stage Reference.vi" "XYZ STAGE USB REFERENCE"() -> (w262:i32)
            n175 = call "PMX-4EX-SA Command Generator.vi"("COMMAND"=commandsnew."constJogPos" ("commands"), "AXIS"=w263) -> ("COMMAND"=w264:string)  [unwired: 13 in]
            n176 = call "sendReceiveCommand.vi"("reference (in)"=w262, "write_string"=w264) -> ()  [unwired: 11 in, 3 out]
          }
          event "OY-": Mouse Up {
            w267 = u16 1 items=["X", "Y", "Z", "U"] ("AXIS")
            n177 = event-data() -> ()  [unwired: 2 out]
            n178 = global read "USB XYZ Stage Reference.vi" "XYZ STAGE USB REFERENCE"() -> (w266:i32)
            n179 = call "PMX-4EX-SA Command Generator.vi"("COMMAND"=commandsnew."stopSlow" ("commands"), "AXIS"=w267) -> ("COMMAND"=w269:string)  [unwired: 13 in]
            n180 = call "sendReceiveCommand.vi"("reference (in)"=w266, "write_string"=w269) -> ()  [unwired: 11 in, 3 out]
          }
        }
        n181 = Wait (ms)(milliseconds to wait=u32 100) -> ()  [unwired: 1 out]
        n182 = Not(x="STOP") -> (.not. x?=w44:bool)
      }
    }
    frame #3 {
      w288 = u16 0 items=["X", "Y", "Z", "U"] ("AXIS")
      w283 = commandsnew."clearErr" ("commands")
      w289 = u16 1 items=["X", "Y", "Z", "U"] ("AXIS")
      w276 = u16 2 items=["X", "Y", "Z", "U"] ("AXIS")
      w277 = u16 2 items=["X", "Y", "Z", "U"] ("AXIS")
      w279 = u16 1 items=["X", "Y", "Z", "U"] ("AXIS")
      w280 = u16 0 items=["X", "Y", "Z", "U"] ("AXIS")
      w278 = commandsnew."powerDown" ("commands")
      n183 = global read "USB XYZ Stage Reference.vi" "XYZ STAGE USB REFERENCE"() -> (w270:i32)
      n184 = call "PMX-4EX-SA Command Generator.vi"("COMMAND"=w278, "AXIS"=w280) -> ("COMMAND"=w295:string)  [unwired: 13 in]
      n185 = call "sendReceiveCommand.vi"("reference (in)"=w270, "write_string"=w295) -> ("reference (out)"=w287:i32, "error out"=w285:errorcluster)  [unwired: 11 in, 1 out]
      n186 = call "PMX-4EX-SA Command Generator.vi"("COMMAND"=w278, "AXIS"=w279) -> ("COMMAND"=w294:string)  [unwired: 13 in]
      n187 = local read "X B"() -> (w297:dbl[unit])
      n188 = local read "Y B"() -> (w296:dbl[unit])
      n189 = call "sendReceiveCommand.vi"("reference (in)"=w287, "write_string"=w294, "error in (no error)"=w285) -> ("reference (out)"=w286:i32, "error out"=w284:errorcluster)  [unwired: 10 in, 1 out]
      n190 = property on="X B" class="DigNum (strict)"("DefVal"=w297) -> ()  [unwired: 2 in, 2 out]
      n191 = property on="Y B" class="DigNum (strict)"("DefVal"=w296) -> ()  [unwired: 2 in, 2 out]
      n192 = call "PMX-4EX-SA Command Generator.vi"("COMMAND"=w278, "AXIS"=w277) -> ("COMMAND"=w293:string)  [unwired: 13 in]
      n193 = call "sendReceiveCommand.vi"("reference (in)"=w286, "write_string"=w293, "error in (no error)"=w284) -> ("reference (out)"=w275:i32)  [unwired: 10 in, 2 out]
      n194 = call "PMX-4EX-SA Command Generator.vi"("COMMAND"=w283, "AXIS"=w288) -> ("COMMAND"=w290:string)  [unwired: 13 in]
      n195 = call "sendReceiveCommand.vi"("reference (in)"=w275, "write_string"=w290) -> ("reference (out)"=w274:i32, "error out"=w282:errorcluster)  [unwired: 11 in, 1 out]
      n196 = call "PMX-4EX-SA Command Generator.vi"("COMMAND"=w283, "AXIS"=w289) -> ("COMMAND"=w291:string)  [unwired: 13 in]
      n197 = call "sendReceiveCommand.vi"("reference (in)"=w274, "write_string"=w291, "error in (no error)"=w282) -> ("reference (out)"=w273:i32, "error out"=w281:errorcluster)  [unwired: 10 in, 1 out]
      n198 = call "PMX-4EX-SA Command Generator.vi"("COMMAND"=w283, "AXIS"=w276) -> ("COMMAND"=w292:string)  [unwired: 13 in]
      n199 = call "sendReceiveCommand.vi"("reference (in)"=w273, "write_string"=w292, "error in (no error)"=w281) -> ("reference (out)"=w272:i32, "error out"=w271:errorcluster)  [unwired: 10 in, 1 out]
      n200 = call "closeDeviceReference.vi"("reference"=w272, "error in (no error)"=w271) -> ()  [unwired: 13 in, 1 out]
    }
  }
  n201 = case shown="False" FALSE {
    frame False {
    }
    frame True {
      n202 = local read "CURRENT LOCATION"() -> (w300:string)
      n203 = local read "DEFINED LOCATIONS"() -> (w303:i32)
      n204 = local read "LOCATIONARRAY"() -> (w304:T3)
      n205 = local read "X"() -> (w302:dbl[unit])
      n206 = local read "Y"() -> (w301:dbl[unit])
      n207 = Bundle("X"=w302, "Y"=w301, "CURRENT LOCATION"=w300) -> (w299:T6)  [unwired: 1 in]
      n208 = Replace Array Subset(array=w304, new element=w299, index=w303) -> (w298:T3)
      n209 = call "sendReceiveCommand.vi"("write_string"="EZ=0") -> ()  [unwired: 12 in, 3 out]
      n210 = local write "LOCATIONARRAY"(w298) -> ()
    }
  }
